vi "Python AE.vi"(0 "connection":refnum<k5>, 1 "error":errorcluster, 3 "run_tcp":bool, 4 "timeout":i32=-1, 7 "u":dbl[][](array[numeric]), 8 "zcomp":dbl format="%#_13g", 10 "Action":T1, 11 "stack":sgl[][](array[numeric])) -> (12 "zcomp out":dbl, 13 "stack out":sgl[][](array[numeric]), 14 "connection out":refnum<k5>, 15 "error out":errorcluster, 16 "u out":dbl[][](array[numeric]), 17 "run_tcp out":bool, 18 "timeout out":i32)   [LabVIEW 2014]
uses:
  Controls/Standard Action.ctl
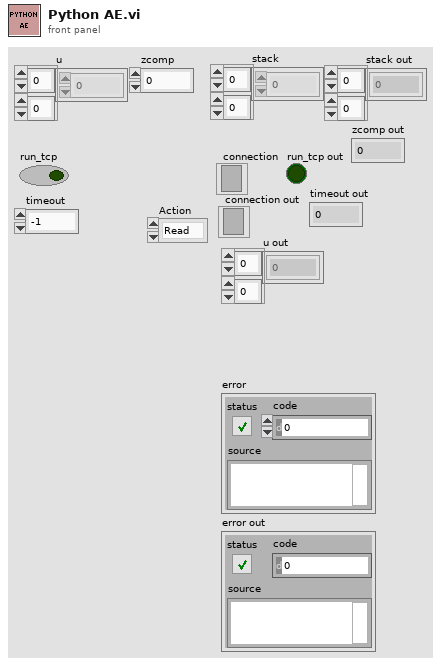
[diagram p1: front panel]
types:
  T1 = typedef "Standard Action.ctl" = enum16{"Read", "Write"}
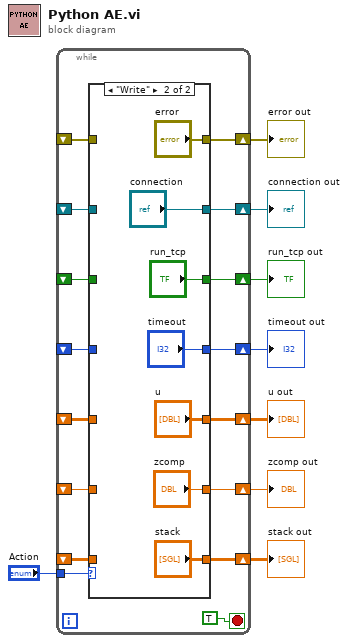
[diagram p0: block diagram]
diagram:
  n1 = while {
    tunnel: "Action" -> [w23]
    shift-right: [w22] -> w7
    shift-left: _ -> [w18]
    shift-right: [w21] -> w6
    shift-left: _ -> [w17]
    shift-right: [w20] -> w5
    shift-left: _ -> [w16]
    shift-right: [w19] -> w4
    shift-left: _ -> [w15]
    shift-right: [w14] -> w3
    shift-left: _ -> [w11]
    shift-right: [w13] -> w2
    shift-left: _ -> [w10]
    shift-right: [w12] -> w1
    shift-left: _ -> [w9]
    stop <- TRUE stop-if-true
    n2 = case shown="\"Write\"" w23 {
      tunnel: [w31 "connection"] -> w22
      tunnel: [w30 "error"] -> w21
      tunnel: [w29 "run_tcp"] -> w20
      tunnel: [w28 "timeout"] -> w19
      tunnel: w18 -> [w31 _]
      tunnel: w17 -> [w30 _]
      tunnel: w16 -> [w29 _]
      tunnel: w15 -> [w28 _]
      tunnel: [w27 "stack"] -> w14
      tunnel: [w26 "u"] -> w13
      tunnel: [w25 "zcomp"] -> w12
      tunnel: w11 -> [w27 _]
      tunnel: w10 -> [w26 _]
      tunnel: w9 -> [w25 _]
      frame "Read", Default {
      }
      frame "Write" {
      }
    }
  }
  "connection out" <- w7
  "error out" <- w6
  "run_tcp out" <- w5
  "timeout out" <- w4
  "stack out" <- w3
  "u out" <- w2
  "zcomp out" <- w1
